vi "Index Group.vi"(8 "error in (no error)":errorcluster, 10 "Group":string, 11 "bt_Blackboard in":refnum<class "Blackboard.lvclass">) -> (0 "error out":errorcluster, 2 "Index":i32, 3 "bt_Blackboard out":refnum<class "Blackboard.lvclass">)   [LabVIEW 2021, in "Blackboard.lvclass"]
uses:
  Blackboard.lvclass
  Blackboard.lvclass/Blackboard.ctl
  Tags Map Type.ctl
  Data Type.ctl
  Status Type.ctl
  Data DVR Type.ctl
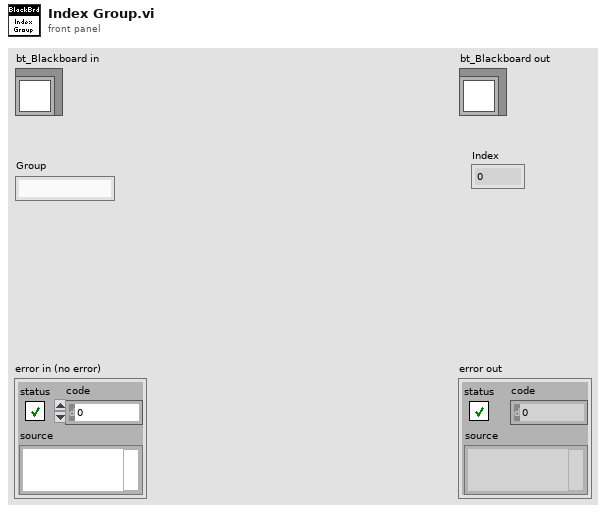
[diagram p1: front panel]
types:
  T1 = typedef "Blackboard.lvclass/Data DVR Type.ctl" = cluster{"Tags":T2, "Status":T3[], "Boolean":bool[], "String":string[], "DBL":dbl[], "SGL":sgl[], "EXT":ext[], "U8":u8[], "U16":u16[], "U32":u32[], "U64":u64[], "I8":i8[], "I16":i16[], "I32":i32[], "I64":i64[], "CDBL":cdb[], "CSGL":csg[], "CEXT":cxt[], "Time":timestamp[], "Variant":variant[], "Waveform":waveform(dbl)[]}
  T2 = typedef "Blackboard.lvclass/Tags Map Type.ctl" = map{string, cluster{"Data Index":i32, "Status Index":i32}}
  T3 = typedef "Blackboard.lvclass/Status Type.ctl" = cluster{"Read?":u32, "Write?":u32, "Data Type":T4}
  T4 = typedef "Blackboard.lvclass/Data Type.ctl" = enum16{"Boolean", "String", "DBL", "SGL", "EXT", "U8", "U16", "U32", "U64", "I8", "I16", "I32", "I64", "CDBL", "CSGL", "CEXT", "Time", "Variant", "Waveform"}
  T5 = typedef "Blackboard.lvclass/Groups Type.ctl" = cluster{"Data":T1[], "Map":T6, "Status":u32[]}
  T6 = typedef "Blackboard.lvclass/Group Map Type.ctl" = map{string, i32}
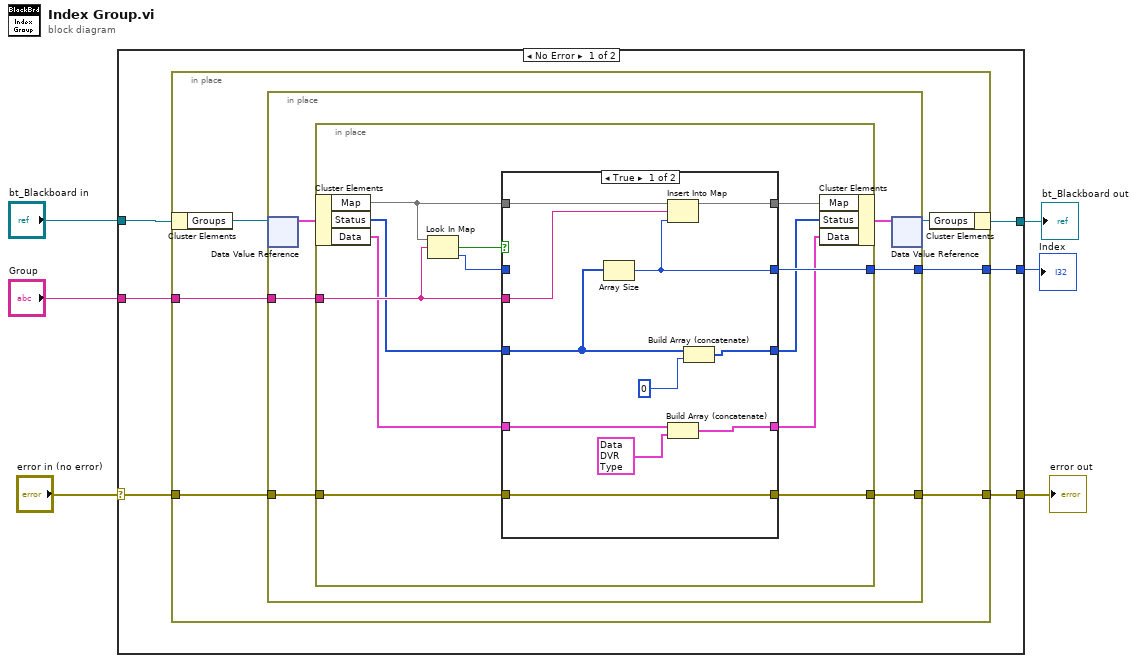
[diagram p0: block diagram]
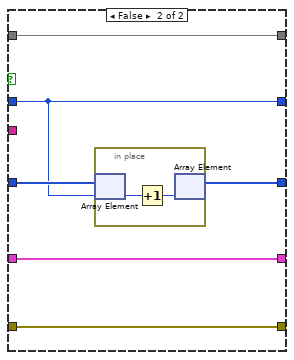
[diagram p2: hidden frame]
diagram:
  n1 = case shown="No Error" "error in (no error)" {
    selector: "error in (no error)" -> [w8 w57]
    tunnel: [w7 w57] -> w5
    tunnel: [w10 w56] -> w3
    tunnel: "bt_Blackboard in" -> [w12 w56]
    tunnel: "Group" -> [w11 _]
    tunnel: [w9 _] -> w1
    frame No Error {
      n2 = in-place {
        in-place-border: w11 -> [w15]
        in-place-border: [w18] -> w9
        in-place-border: w8 -> [w17]
        in-place-border: [w16] -> w7
        n3 = in-place-cluster #1(w12) -> ("Groups"=w14:refnum<data-value>)
        n4 = in-place {
          in-place-border: [w24] -> w18
          in-place-border: w17 -> [w23]
          in-place-border: [w22] -> w16
          in-place-border: w15 -> [w21]
          n5 = in-place-dvr #2(w14) -> (w20:T5)  [unwired: 1 out]
          n6 = in-place {
            in-place-border: [w36] -> w24
            in-place-border: w23 -> [w35]
            in-place-border: [w34] -> w22
            in-place-border: w21 -> [w33]
            n7 = in-place-cluster #3(w20) -> ("Map"=w30:T6, "Status"=w28:u32[], "Data"=w26:T1[])
            n8 = Look In Map(map=w30, key=w33) -> (key not found?=w32:bool, value=w31:i32)  [unwired: 1 in]
            n9 = case shown="True" w32 {
              tunnel: w33 -> [w41 _]
              tunnel: [w39 w49] -> w36
              tunnel: w28 -> [w40 w53]
              tunnel: [w47 w52] -> w27
              tunnel: w26 -> [w45 w51]
              tunnel: [w44 w51] -> w25
              tunnel: w35 -> [w38 w50]
              tunnel: [w38 w50] -> w34
              tunnel: w30 -> [w43 w48]
              tunnel: [w42 w48] -> w29
              tunnel: w31 -> [_ w49]
              frame True {
                n10 = Array Size(array=w40) -> (size(s)=w39:i32)
                n11 = Insert Into Map(map in=w43, key=w41, value=w39) -> (map out=w42:T6)  [unwired: 2 out]
                n12 = Build Array (concatenate)(w45, T1 {"Tags"={}, "Status"=[], "Boolean"=[], "String"=[], "DBL"=[], "SGL"=[], "EXT"=[], "U8"=[], "U16"=[], "U32"=[], "U64"=[], "I8"=[], "I16"=[], "I32"=[], "I64"=[], "CDBL"=[], "CSGL"=[], "CEXT"=[], "Time"=[], "Variant"=[], "Waveform"=[]} ("Data")) -> (w44:T1[])
                n13 = Build Array (concatenate)(w40, u32 0) -> (w47:u32[])
              }
              frame False {
                n14 = in-place {
                  n15 = in-place-array #4(w53, w49) -> (w55:u32)
                  n16 = Increment(x=w55) -> (x+1=w54:u32)
                  n17 = in-place-array #4(w54) -> (w52:u32[])  [unwired: 1 out]
                }
              }
            }
            n18 = in-place-cluster #3("Map"=w29, "Status"=w27, "Data"=w25) -> (w19:T5)
          }
          n19 = in-place-dvr #2(w19) -> (w13:refnum<data-value>)  [unwired: 1 out]
        }
        n20 = in-place-cluster #1("Groups"=w13) -> (w10:refnum<class "Blackboard.lvclass">)
      }
    }
    frame Error {
    }
  }
  "error out" <- w5
  "bt_Blackboard out" <- w3
  "Index" <- w1
